vi "PH Cross Correlation.vi"(10 "Digest 2":cluster{"*id":u32, "*Coeffs":u32, "size":i32}, 11 "Digest 1":cluster{"*id":u32, "*Coeffs":u32, "size":i32}) -> (3 "Perceptual Cross Correlation":dbl)   [LabVIEW 2020, in "Perceptual Hash Comparison.lvclass"]
uses:
  Perceptual Hash Comparison.lvclass
  phash DLL/pHash.dll
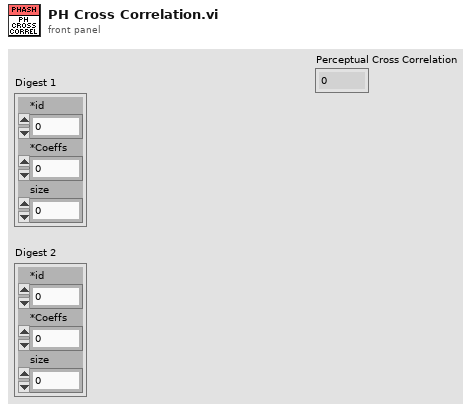
[diagram p1: front panel]
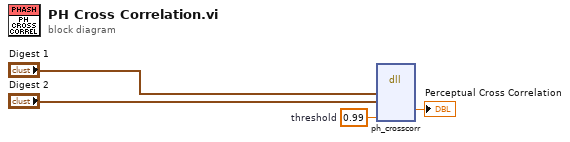
[diagram p0: block diagram]
diagram:
  w2 = 0.99  # threshold
  n1 = dll-call lib="D:/code/labview/labview-reddit-coding-challenge-june-2021/Perceptual Hash Comparison/phash DLL/pHash.dll" fn="ph_crosscorr"("x"="Digest 1", "y"="Digest 2", "threshold"=w2) -> ("pcc"=→"Perceptual Cross Correlation":dbl)  [unwired: 8 in, 2 out]
